vi "IMAQ-MWT Contour SPINE TEST (HOST).vi"() -> ()   [LabVIEW 2015]
uses:
  <vilib>/FPGAPlugInAG/PCIe-1473R-LX110/niLvFpga_Open_PCIe-1473R-LX110.vi
  <vilib>/rvi/interface/common/dynamic/niFpgaDynamicAddResources.vi
  <vilib>/rvi/interface/common/niFpgaWaitOnOcc.vi
  <vilib>/Utility/error.llb/Error Cluster From Error Code.vi
  <vilib>/rvi/errors/niLvFpgaAdjustHostInterfaceError.vi
  <vilib>/FPGAPlugInAG/Dynamic/niLvFpga_Close_Dynamic.vi
  <vilib>/rvi/interface/nirviOpenFPGA/nirviOpenFPGA.xnode
  FPGA Bitfiles/IMAQ(MWT)_FPGATarget_IMAQ-MWTContourS_6I5mIhXKFac.lvbitx
  <vilib>/rvi/interface/nirviMethod/nirviMethod.xnode
  <vilib>/rvi/interface/nirviReadWriteControl/nirviReadWriteControl.xnode
  <vilib>/rvi/interface/nirviCloseFPGA/nirviCloseFPGA.xnode
  <vilib>/rvi/errors/niLvFpgaMergeErrorWithErrorCode.vi
  <vilib>/FPGAPlugInAG/Dynamic/niLvFpga_ReadFifo_Dynamic.vi
  <vilib>/FPGAPlugInAG/Dynamic/niLvFpga_ConfigureFifo_Dynamic.vi
  <vilib>/FPGAPlugInAG/Dynamic/niLvFpga_StartFifo_Dynamic.vi
  <vilib>/FPGAPlugInAG/Dynamic/niLvFpga_WriteFifo_Dynamic.vi
  NiFpgaLv.dll
  <vilib>/rvi/interface/Simulation/niFpgaSimulationCallBeginRW.vi
panel:
  out "Edge Image":T1(plugin-control)
  in  "Low":u8=100
  in  "High":u8=255
  out "BWImage":T1(plugin-control)
  out "Raw Image":T1(plugin-control)
  in  "Frame #":i32=40
  out "Contour/SPINE":cluster{u16[], u16[]}[](graph)
  out "Frame Count":i32
  in  "Loop Interval":u32=1000
  in  "Stop Button":bool
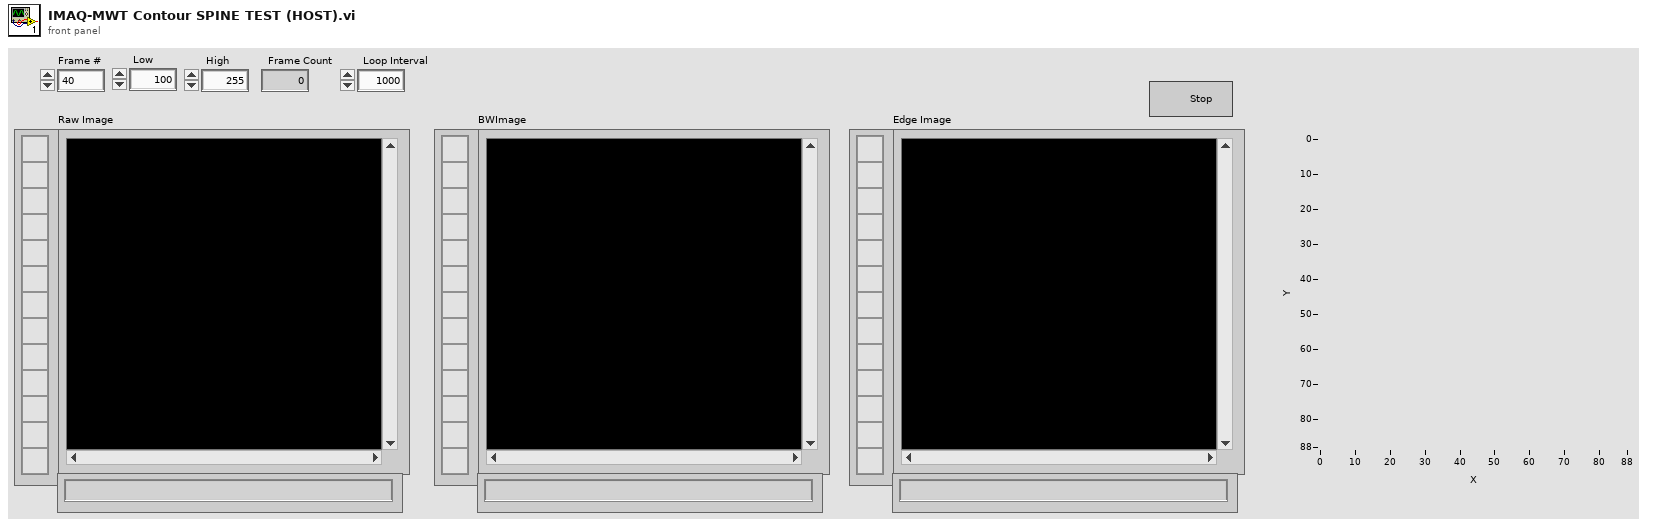
[diagram p1: front panel]
types:
  T1 = typedef "IMAQ Image.ctl" = refnum<image>
  T2 = enum16{"big-endian, network order", "native, host order", "little-endian"}
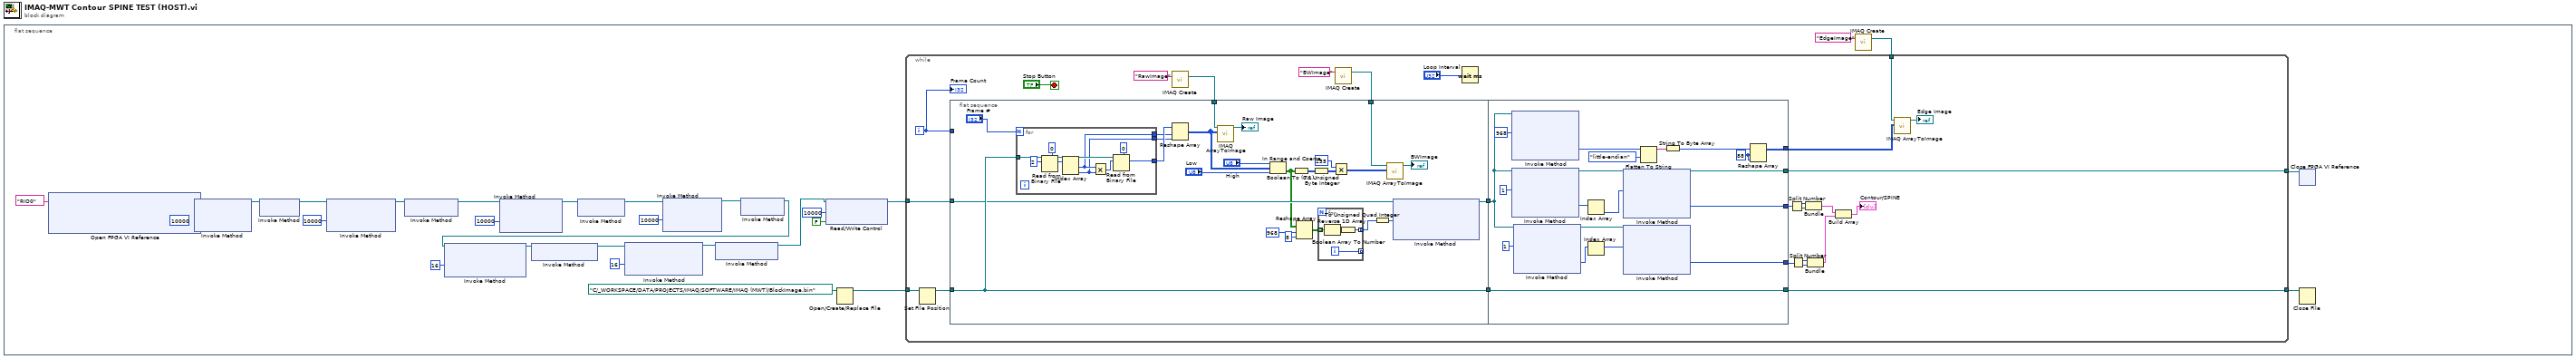
[diagram p0: block diagram]
diagram:
  n1 = flat-sequence {
    frame #0 {
      n2 = xnode "Open FPGA VI Reference"("resource name"=tag "RIO0") -> ("FPGA VI Reference Out"=w24:refnum<k20>)  [unwired: 1 in, 1 out]
      n3 = xnode "Invoke Method"("FPGA VI Reference In"=w24, "Requested Depth"=u32 10000) -> ("FPGA VI Reference Out"=w22:refnum<k20>)  [unwired: 1 in, 2 out]
      n4 = xnode "Invoke Method"("FPGA VI Reference In"=w22) -> ("FPGA VI Reference Out"=w19:refnum<k20>)  [unwired: 1 in, 1 out]
      n5 = xnode "Invoke Method"("FPGA VI Reference In"=w19, "Requested Depth"=u32 10000) -> ("FPGA VI Reference Out"=w21:refnum<k20>)  [unwired: 1 in, 2 out]
      n6 = xnode "Invoke Method"("FPGA VI Reference In"=w21) -> ("FPGA VI Reference Out"=w14:refnum<k20>)  [unwired: 1 in, 1 out]
      n7 = xnode "Invoke Method"("FPGA VI Reference In"=w14, "Requested Depth"=u32 10000) -> ("FPGA VI Reference Out"=w15:refnum<k20>)  [unwired: 1 in, 2 out]
      n8 = xnode "Invoke Method"("FPGA VI Reference In"=w15) -> ("FPGA VI Reference Out"=w7:refnum<k20>)  [unwired: 1 in, 1 out]
      n9 = xnode "Invoke Method"("FPGA VI Reference In"=w7, "Requested Depth"=u32 10000) -> ("FPGA VI Reference Out"=w6:refnum<k20>)  [unwired: 1 in, 2 out]
      n10 = xnode "Invoke Method"("FPGA VI Reference In"=w6) -> ("FPGA VI Reference Out"=w4:refnum<k20>)  [unwired: 1 in, 1 out]
      n11 = xnode "Invoke Method"("FPGA VI Reference In"=w4, "Requested Depth"=u32 16) -> ("FPGA VI Reference Out"=w12:refnum<k20>)  [unwired: 1 in, 2 out]
      n12 = xnode "Invoke Method"("FPGA VI Reference In"=w12) -> ("FPGA VI Reference Out"=w8:refnum<k20>)  [unwired: 1 in, 1 out]
      n13 = xnode "Invoke Method"("FPGA VI Reference In"=w8, "Requested Depth"=u32 16) -> ("FPGA VI Reference Out"=w3:refnum<k20>)  [unwired: 1 in, 2 out]
      n14 = xnode "Invoke Method"("FPGA VI Reference In"=w3) -> ("FPGA VI Reference Out"=w2:refnum<k20>)  [unwired: 1 in, 1 out]
      n15 = xnode "Read/Write Control"("FPGA VI Reference In"=w2, "Clock Cycles Limit"=u32 10000, "TP"=FALSE) -> ("FPGA VI Reference Out"=w18:refnum<k20>)  [unwired: 1 in, 1 out]
      n16 = Open/Create/Replace File(file path (use dialog)=path "C:/_WORKSPACE/DATA/PROJECTS/IMAQ/SOFTWARE/IMAQ (MWT)/BlockImage.bin") -> (refnum out=w27:refnum<file>)  [unwired: 5 in, 2 out]
      n17 = call "IMAQ Create"("Image Name"="EdgeImage") -> ("New Image"=w9:T1)  [unwired: 4 in, 1 out]
      n18 = while {
        tunnel: w18 -> [w55]
        tunnel: [w54] -> w28
        tunnel: w27 -> [w52]
        tunnel: [w47] -> w26
        tunnel: w9 -> [w43]
        i -> [w37]
        stop <- "Stop Button" stop-if-true
        n19 = Set File Position(refnum=w52) -> (refnum out=w49:refnum<file>)  [unwired: 3 in, 1 out]
        n20 = flat-sequence {
          tunnel: [w79] -> w50
          tunnel: [w78] -> w48
          tunnel: w40 -> [w71]
          tunnel: w49 -> [w78]
          tunnel: w55 -> [w77]
          tunnel: w38 -> [w62]
          tunnel: w37 -> [_]
          tunnel: [w112] -> w54
          tunnel: w50 -> [w106]
          tunnel: [w110] -> w36
          tunnel: [w101] -> w44
          tunnel: [w105] -> w47
          tunnel: w48 -> [w105]
          tunnel: [w96] -> w33
          frame #0 {
            n21 = for {
              N: "Frame #" -> [_]
              tunnel: w78 -> [w93]
              tunnel: [w87] -> w75
              tunnel: [w85] -> w74
              tunnel: [w84] -> w73
              n22 = Read from Binary File(5:0 ("count (1)"), 10:2 ("count (1)"), 11:w93) -> (2:w89:i32[], 3:w91:refnum<file>)  [unwired: 3 in, 2 out]
              n23 = Index Array(array=w89) -> (element #1=w85:i32, element #2=w84:i32)  [unwired: 2 in]
              n24 = Multiply(x=w85, y=w84) -> (x*y=w86:i32)
              n25 = Read from Binary File(5:u8 0 ("count (1)"), 10:w86, 11:w91) -> (2:w87:u8[])  [unwired: 3 in, 3 out]
            }
            n26 = Reshape Array(w75, w74, w73) -> (w70:u8[][])
            n27 = call "IMAQ ArrayToImage"("Image Pixels (U8)"=w70, "Image"=w71) -> ("Image Out"=→"Raw Image":T1)  [unwired: 8 in, 1 out]
            n28 = In Range and Coerce(upper limit="High", x=w70, lower limit="Low") -> (In Range?=w61:bool[][])  [unwired: 1 out]
            n29 = Boolean To (0,1)(Boolean=w61) -> (0, 1=w67:i16[][])
            n30 = Reshape Array(w61, 968 ("dimension size"), 8 ("dimension size")) -> (w58:bool[][])
            n31 = To Unsigned Byte Integer(number=w67) -> (unsigned 8bit integer=w66:u8[][])
            n32 = for {
              tunnel: w58 -> [w81] mode=indexing
              tunnel: [w83] -> w57 mode=indexing
              tunnel: [w82] -> _ mode=indexing
              i -> [w82]
              n33 = Reverse 1D Array(array=w81) -> (reversed array=w80:bool[])
              n34 = Boolean Array To Number(Boolean array=w80) -> (number=w83:u32)
            }
            n35 = Multiply(x=u8 255 ("count (1)"), y=w66) -> (x*y=w63:u8[][])
            n36 = To Unsigned Quad Integer(1:w57) -> (0:w76:u64[])
            n37 = call "IMAQ ArrayToImage"("Image Pixels (U8)"=w63, "Image"=w62) -> ("Image Out"=→"BWImage":T1)  [unwired: 8 in, 1 out]
            n38 = xnode "Invoke Method"("FPGA VI Reference In"=w77, "Data"=w76) -> ("FPGA VI Reference Out"=w79:refnum<k20>)  [unwired: 2 in, 2 out]
          }
          frame #1 {
            w100 = 88 ("dimension size")
            n39 = xnode "Invoke Method"("FPGA VI Reference In"=w106, "Number of Elements"=u32 1) -> ("FPGA VI Reference Out"=w111:refnum<k20>, "Data"=w108:u32[])  [unwired: 2 in, 2 out]
            n40 = xnode "Invoke Method"("FPGA VI Reference In"=w106, "Number of Elements"=u32 968) -> ("Data"=w104:u64[])  [unwired: 2 in, 3 out]
            n41 = xnode "Invoke Method"("FPGA VI Reference In"=w106, "Number of Elements"=u32 1) -> ("FPGA VI Reference Out"=w98:refnum<k20>, "Data"=w95:u32[])  [unwired: 2 in, 2 out]
            n42 = Index Array(array=w108) -> (element=w107:u32)  [unwired: 1 in]
            n43 = Index Array(array=w95) -> (element=w94:u32)  [unwired: 1 in]
            n44 = xnode "Invoke Method"("FPGA VI Reference In"=w111, "Number of Elements"=w107) -> ("FPGA VI Reference Out"=w112:refnum<k20>, "Data"=w110:u32[])  [unwired: 2 in, 2 out]
            n45 = xnode "Invoke Method"("FPGA VI Reference In"=w98, "Number of Elements"=w94) -> ("Data"=w96:u32[])  [unwired: 2 in, 3 out]
            n46 = Flatten To String(anything=w104, byte order (0:big-endian, network order)=T2."little-endian") -> (data string=w102:string)  [unwired: 2 in, 2 out]
            n47 = String To Byte Array(string=w102) -> (unsigned byte array=w103:u8[])
            n48 = Reshape Array(w103, w100, w100) -> (w101:u8[][])
          }
        }
        n49 = call "IMAQ Create"("Image Name"="RawImage") -> ("New Image"=w40:T1)  [unwired: 4 in, 1 out]
        n50 = call "IMAQ Create"("Image Name"="BWImage") -> ("New Image"=w38:T1)  [unwired: 4 in, 1 out]
        n51 = Wait (ms)(milliseconds to wait="Loop Interval") -> ()  [unwired: 1 out]
        n52 = Split Number(x=w36) -> (hi(x)=w46:u16[], lo(x)=w45:u16[])
        n53 = Split Number(x=w33) -> (hi(x)=w34:u16[], lo(x)=w35:u16[])
        n54 = Bundle(w46, w45) -> (w32:cluster{u16[], u16[]})  [unwired: 1 in]
        n55 = Bundle(w34, w35) -> (w30:cluster{u16[], u16[]})  [unwired: 1 in]
        n56 = Build Array(w32, w30) -> (→"Contour/SPINE":cluster{u16[], u16[]}[])
        n57 = call "IMAQ ArrayToImage"("Image Pixels (U8)"=w44, "Image"=w43) -> ("Image Out"=→"Edge Image":T1)  [unwired: 8 in, 1 out]
        "Frame Count" <- w37
      }
      n58 = xnode "Close FPGA VI Reference"("FPGA VI Reference In"=w28) -> ()  [unwired: 1 in, 1 out]
      n59 = Close File(refnum=w26) -> ()  [unwired: 1 in, 2 out]
    }
  }
